vi "Acquire.vi"(8 "error in (no error)":errorcluster caption="错误输入（无错误）", 9 "Data Queue":refnum<queue> caption="数据队列", 10 "Data Notifier":refnum<notifier> caption="数据通知器", 11 "Hardware Resources in":T1={"PLC设置"={"端口选择"="COM3", "波特率"=0, "校检"=0, "数据位"=0}, "动作设置"={"自动跳法测试动作"={"夹紧"={"PLC指令"={"变量类型"=2, "PLC地址"="0", "16位/32位"=0, "写入数据(写入时有效)"=""}}, "分中"={}, "通油"={"打开主阀"={"变量类型"=2, "PLC地址"="0", "16位/32位"=0, "写入数据(写入时有效)"=""}, "打开电磁阀"={"变量类型"=2, "PLC地址"="0", "16位/32位"=0, "写入数据(写入时有效)"=""}}, "自动对中"={}, "内泄漏测试"={}, "压销"={"PLC指令"={"变量类型"=2, "PLC地址"="0", "16位/32位"=0, "写入数据(写入时有效)"=""}}}}} caption="硬件资源输入" {"动作设置"."自动跳法测试动作"."压销"."PLC指令"."16位/32位" items=["16bit", "32bit"]; "动作设置"."自动跳法测试动作"."压销"."PLC指令"."变量类型" items=["X", "Y", "M", "D"]; "动作设置"."自动跳法测试动作"."通油"."打开电磁阀"."16位/32位" items=["16bit", "32bit"]; "动作设置"."自动跳法测试动作"."通油"."打开电磁阀"."变量类型" items=["X", "Y", "M", "D"]; "动作设置"."自动跳法测试动作"."通油"."打开主阀"."16位/32位" items=["16bit", "32bit"]; "动作设置"."自动跳法测试动作"."通油"."打开主阀"."变量类型" items=["X", "Y", "M", "D"]; "动作设置"."自动跳法测试动作"."夹紧"."PLC指令"."16位/32位" items=["16bit", "32bit"]; "动作设置"."自动跳法测试动作"."夹紧"."PLC指令"."变量类型" items=["X", "Y", "M", "D"]; "PLC设置"."数据位" items=["7"=7, "8"=8]; "PLC设置"."校检" items=["无", "偶", "奇"]; "PLC设置"."波特率" items=["9600"=9600, "19200"=19200, "115200"=115200]}) -> (0 "error out":errorcluster caption="错误输出", 3 "Hardware Resources out":T1={"PLC设置"={"端口选择"="COM3", "波特率"=0, "校检"=0, "数据位"=0}, "动作设置"={"自动跳法测试动作"={"夹紧"={"PLC指令"={"变量类型"=2, "PLC地址"="0", "16位/32位"=0, "写入数据(写入时有效)"=""}}, "分中"={}, "通油"={"打开主阀"={"变量类型"=2, "PLC地址"="0", "16位/32位"=0, "写入数据(写入时有效)"=""}, "打开电磁阀"={"变量类型"=2, "PLC地址"="0", "16位/32位"=0, "写入数据(写入时有效)"=""}}, "自动对中"={}, "内泄漏测试"={}, "压销"={"PLC指令"={"变量类型"=2, "PLC地址"="0", "16位/32位"=0, "写入数据(写入时有效)"=""}}}}} caption="硬件资源输出" {"动作设置"."自动跳法测试动作"."压销"."PLC指令"."16位/32位" items=["16bit", "32bit"]; "动作设置"."自动跳法测试动作"."压销"."PLC指令"."变量类型" items=["X", "Y", "M", "D"]; "动作设置"."自动跳法测试动作"."通油"."打开电磁阀"."16位/32位" items=["16bit", "32bit"]; "动作设置"."自动跳法测试动作"."通油"."打开电磁阀"."变量类型" items=["X", "Y", "M", "D"]; "动作设置"."自动跳法测试动作"."通油"."打开主阀"."16位/32位" items=["16bit", "32bit"]; "动作设置"."自动跳法测试动作"."通油"."打开主阀"."变量类型" items=["X", "Y", "M", "D"]; "动作设置"."自动跳法测试动作"."夹紧"."PLC指令"."16位/32位" items=["16bit", "32bit"]; "动作设置"."自动跳法测试动作"."夹紧"."PLC指令"."变量类型" items=["X", "Y", "M", "D"]; "PLC设置"."数据位" items=["7"=7, "8"=8]; "PLC设置"."校检" items=["无", "偶", "奇"]; "PLC设置"."波特率" items=["9600"=9600, "19200"=19200, "115200"=115200]})   [LabVIEW 2015, in "Action.lvlib"]
doc: "执行采集。替换程序框图的内容，添加对采集硬件的调用。"
uses:
  Action.lvlib
  <vilib>/DAQmx/read.llb/DAQmx Read (Analog 1D Wfm NChan NSamp).vi
  <resource>/objmgr/daqmx.rc
  Hardware Configuration.ctl
  PLC/PLC.lvlib
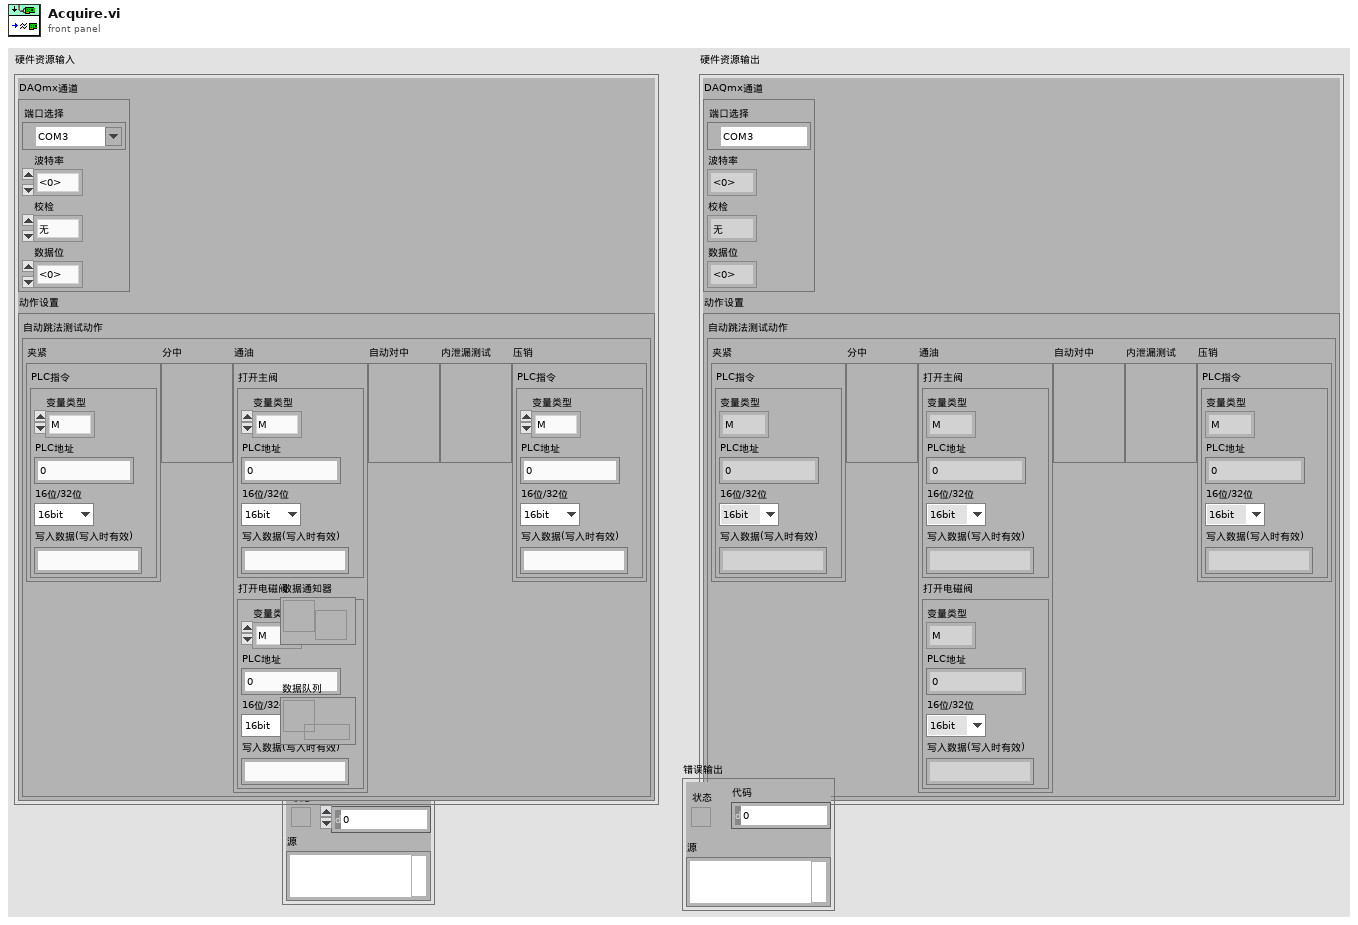
[diagram p1: front panel]
types:
  T1 = typedef "Action.lvlib/Hardware Configuration.ctl" = cluster{"PLC设置":T2, "动作设置":T3}
  T2 = typedef "PLC.lvlib/PLC设置.ctl" = cluster{"端口选择":refnum<visa-resource-name>, "波特率":u32, "校检":u32, "数据位":u32}
  T3 = typedef "Action.lvlib/动作设置.ctl" = cluster{"自动跳法测试动作":T4}
  T4 = typedef "Action.lvlib/自动调阀测试动作设置.ctl" = cluster{"夹紧":cluster{"PLC指令":T5}, "分中":cluster{}, "通油":cluster{"打开主阀":T5, "打开电磁阀":T5}, "自动对中":cluster{}, "内泄漏测试":cluster{}, "压销":cluster{"PLC指令":T5}}
  T5 = typedef "PLC.lvlib/PLC指令.ctl" = cluster{"变量类型":u32, "PLC地址":string, "16位/32位":u32, "写入数据(写入时有效)":string}
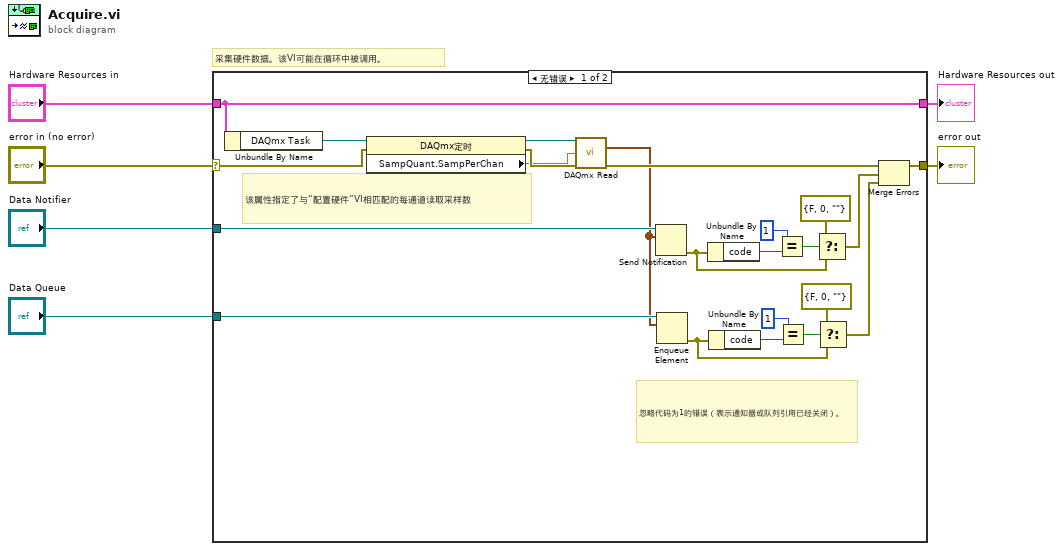
[diagram p0: block diagram]
diagram:
  # "采集硬件数据。该VI可能在循环中被调用。"
  n1 = case shown="无错误" "error in (no error)" {
    selector: "error in (no error)" -> [w9 w30]
    tunnel: [w29 w30] -> w5
    tunnel: "Hardware Resources in" -> [w14 w31]
    tunnel: [w14 w31] -> w3
    tunnel: "Data Notifier" -> [w28 _]
    tunnel: "Data Queue" -> [w15 _]
    frame No Error {
      # "该属性指定了与“配置硬件”VI相匹配的每通道读取采样数"
      # "忽略代码为1的错误（表示通知器或队列引用已经关闭）。"
      n2 = Unbundle By Name(w14) -> ("DAQmx Task"=w11:refnum<k21>)
      n3 = property class="DAQmx定时"(reference=w11, error in=w9) -> (reference out=w10:refnum<k21>, error out=w8:errorcluster, "SampQuant.SampPerChan"=w7:dbl)
      n4 = call-poly <vilib>:"DAQmx Read.vi"("task/channels in"=w10, "number of samples per channel"=w7, "error in"=w8) -> ("data"=w12:waveform(dbl)[], "error out"=w13:errorcluster)  [unwired: 10 in, 1 out]
      n5 = Send Notification(notification=w12, notifier=w28) -> (error out=w24:errorcluster)  [unwired: 1 in, 1 out]
      n6 = Enqueue Element(queue=w15, element=w12) -> (error out=w20:errorcluster)  [unwired: 2 in, 2 out]
      n7 = Unbundle By Name(w24) -> ("code"=w27:i32)
      n8 = Unbundle By Name(w20) -> ("code"=w17:i32)
      n9 = Equal?(x=1, y=w27) -> (x = y?=w25:bool)
      n10 = Equal?(x=1, y=w17) -> (x = y?=w19:bool)
      n11 = Select(t=errorcluster {"status"=FALSE, "code"=0, "source"=""} ("error constant"), s=w25, f=w24) -> (s? t:f=w23:errorcluster)
      n12 = Select(t=errorcluster {"status"=FALSE, "code"=0, "source"=""} ("error constant"), s=w19, f=w20) -> (s? t:f=w16:errorcluster)
      n13 = Merge Errors(w13, w23, w16) -> (w29:errorcluster)
    }
    frame Error {
    }
  }
  "Hardware Resources out" <- w3
  "error out" <- w5
